vi "OOK_TEST.vi"() -> ()   [LabVIEW 2014]
panel:
  in  "trigger level":dbl
  in  "downsampling factor":i32
  in  "upsampling number":i32
  in  "String":string="如果采用顺序流接收的方式：先从USRP缓存区获取数据，分局数据确定物理层分组，再将分组传给下面的解调模块。由于解码耗时较长，会拖累获取数据的速度，使得从USRP缓存区获取数据的速率低于采样率，从而引发缓冲区爆满的问题。\n那么将接收和解调使用并行运行的方式：一个线程获取缓存区数据，并根据信号强度抽取出一个物理层分组，将分组放到共享队列里面；另一个线程监听该队列，一旦获取一个分组，就进行解调和解码。这种方式可以有效地解决缓存区爆满的问题。\n我真是太TM机制了"
  out "string 2":string
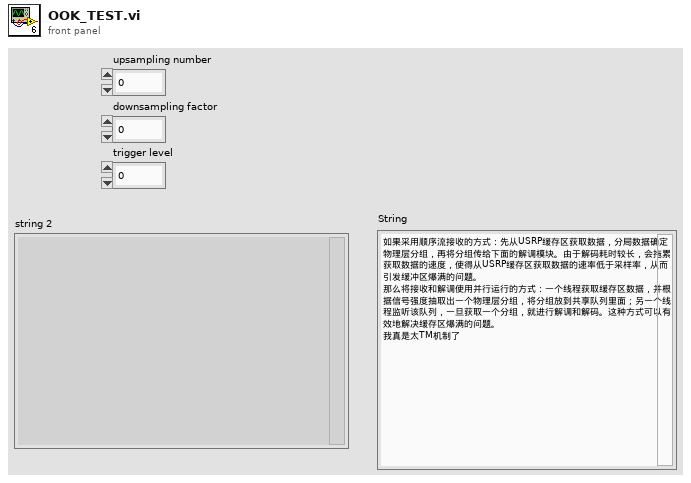
[diagram p1: front panel]
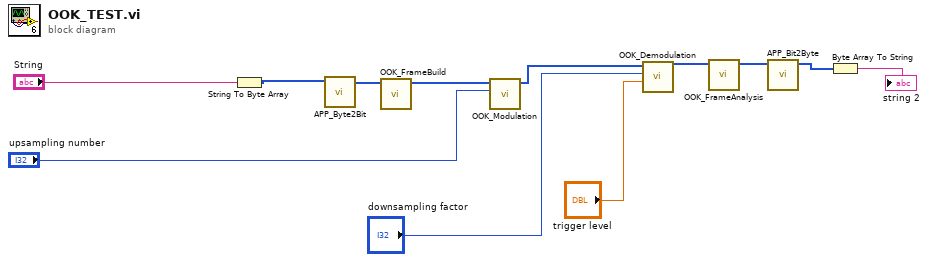
[diagram p0: block diagram]
diagram:
  n1 = String To Byte Array(string="String") -> (unsigned byte array=w7:u8[])
  n2 = call "APP_Byte2Bit.vi"("input byte stream"=w7) -> ("output bit stream"=w5:i8[])  [unwired: 10 in]
  n3 = call "OOK_FrameBuild.vi"("input bit stream"=w5) -> ("output bit stream"=w8:i8[])  [unwired: 10 in]
  n4 = call "OOK_Modulation.vi"("upsampling number"="upsampling number", "input bit stream"=w8) -> ("output bit stream"=w3:i8[])  [unwired: 9 in]
  n5 = call "OOK_Demodulation.vi"("trigger level"="trigger level", "downsampling factor"="downsampling factor", "input symbol stream"=w3) -> ("output bit stream"=w10:i8[])  [unwired: 8 in]
  n6 = call "OOK_FrameAnalysis.vi"("input bit stream"=w10) -> ("data bit stream"=w9:i8[])  [unwired: 10 in]
  n7 = call "APP_Bit2Byte.vi"("input bit stream"=w9) -> ("output byte stream"=w12:u8[])  [unwired: 10 in]
  n8 = Byte Array To String(unsigned byte array=w12) -> (string=→"string 2":string)
